vi "Upload Configuration Files to PXI.vi"(8 "error in":errorcluster, 10 "Destination":string="C:\\ni-rt\\fsuarez", 11 "PXI IP":string="192.168.0.4") -> (0 "error out":errorcluster)   [LabVIEW 2013]
doc: "This VI sends all the files in the Host PC located at \"mf3_labview\\Configuration Files\" to the PXI.\n\nYou just need to run it!"
uses:
  <vilib>/FTP/NI_FTP.lvlib
panel:
  # "This VI sends all the files in the Host PC located at \n\"grips_labview\\Projects\\Configuration Files\" to the \nPXI.\n\nYou just need to run it!"
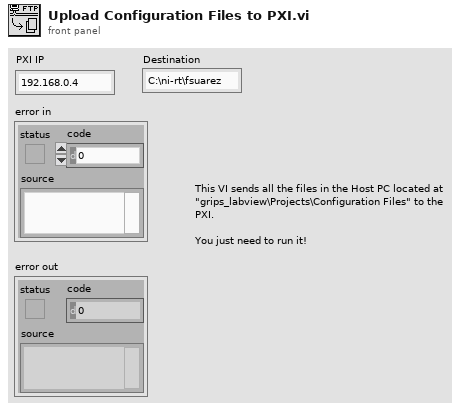
[diagram p1: front panel]
types:
  T1 = cluster{"remote path":string, "local path":path, "binary":bool, "data":string}
  T2 = typedef "NI_FTP.lvlib/FTP Session.ctl" = refnum<k5>
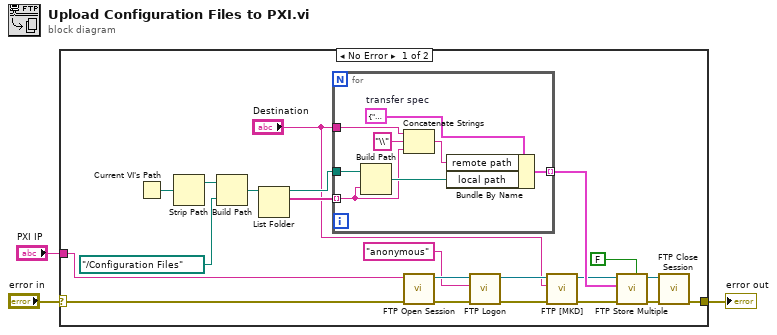
[diagram p0: block diagram]
diagram:
  n1 = case shown="No Error" "error in" {
    selector: "error in" -> [w5 w33]
    tunnel: [w11 w33] -> w3
    tunnel: "PXI IP" -> [w4 _]
    frame No Error {
      n2 = Current VI's Path() -> (path=w20:path)
      n3 = Strip Path(path=w20) -> (stripped path=w19:path)  [unwired: 1 out]
      n4 = Build Path(base path=w19, name or relative path=path "../Configuration Files" ("Relative Path to be Sent")) -> (appended path=w18:path)
      n5 = List Folder(path=w18) -> (path out=w17:path, filenames=w16:string[])  [unwired: 3 in, 2 out]
      n6 = for {
        tunnel: w17 -> [w32]
        tunnel: w16 -> [w26] mode=indexing
        tunnel: [w29] -> w13 mode=indexing
        tunnel: "Destination" -> [w27]
        w31 = T1 {"remote path"="", "local path"=path "", "binary"=FALSE, "data"=""}  # transfer spec
        n7 = Build Path(base path=w32, name or relative path=w26) -> (appended path=w28:path)
        n8 = Concatenate Strings(w27, "\\" ("user"), w26) -> (w30:string)
        n9 = Bundle By Name(cluster=w31, "remote path"=w30, "local path"=w28) -> (w29:T1)
      }
      n10 = call <vilib>:"FTP Open Session.vi"("error in (no error)"=w5, "address"=w4) -> ("error out"=w22:errorcluster, "ftp session"=w24:T2)  [unwired: 6 in, 2 out]
      n11 = call <vilib>:"FTP Logon.vi"("error in (no error)"=w22, "user"="anonymous", "ftp session"=w24) -> ("error out"=w9:errorcluster, "ftp session out"=w10:T2)  [unwired: 5 in, 2 out]
      n12 = call <vilib>:"FTP [MKD].vi"("error in (no error)"=w9, "directory path"="Destination", "ftp session"=w10) -> ("error out"=w6:errorcluster, "ftp session out"=w7:T2)  [unwired: 5 in, 2 out]
      n13 = call <vilib>:"FTP Store Multiple.vi"("active (T)"=FALSE, "error in (no error)"=w6, "file specifications"=w13, "ftp session"=w7) -> ("error out"=w14:errorcluster, "ftp session out"=w15:T2)  [unwired: 5 in, 1 out]
      n14 = call <vilib>:"FTP Close Session.vi"("error in (no error)"=w14, "ftp session"=w15) -> ("error out"=w11:errorcluster)  [unwired: 6 in, 3 out]
    }
    frame Error {
    }
  }
  "error out" <- w3
